vi "geis.vi"(3 "Draw":T2(ring), 7 "DLLPath":path, 8 "error in (no error)":errorcluster, 9 "GEIS Parameters":T3={"Step_number"=0, "Initial_Current_step"=0.0, "vs_initial "=TRUE, "Final_Current_step"=0.001, "vs_final"=TRUE, "Duration_step"=1.0, "Record_every_dE"=0.1, "Record_every_dT"=0.1, "Initial_frequency"=100000.0, "sweep"=FALSE, "Final_frequency"=1.0, "Frequency_number"=51, "Amplitude_Current"=0.001, "Wait_for_steady"=2.0, "Average_N_times"=1, "Correction"=TRUE, "I_Range"=7, "Bandwidth"=5, "em"=1, "ce"=0} {"ce" items=["Standard", "CE to ground"]; "em" max=10 format="%.5f"; "Initial_Current_step" min=-10 max=10 format="%.5f"; "Step_number" min=0 step=1; "I_Range" items=["1pA", "1nA", "10nA", "100nA", "1µA", "10µA", "100µA", "1mA", "10mA", "100mA", "1A", "Booster", "Auto"]; "Bandwidth" items=["1"=1, "2"=2, "3"=3, "4"=4, "5"=5, "6"=6, "7"=7, "8"=8, "9"=9]; "Wait_for_steady" min=0 format="%.2f"; "Record_every_dT" min=0 format="%.2e"; "Record_every_dE" min=0 format="%.2e"; "Duration_step" min=0 format="%.5f"; "Final_Current_step" min=-10 max=10 format="%.5f"; "Average_N_times" min=1 max=1000 step=1; "Amplitude_Current" min=0 max=100 format="%.2e"; "Final_frequency" min=1e-05 max=1000000 format="%.2e"; "Frequency_number" min=1 max=10000; "Initial_frequency" min=1e-05 max=1000000 format="%.2e"}, 10 "Channel":u8(ring) items=["1", "2", "3", "4", "5", "6", "7", "8", "9", "10", "11", "12", "13", "14", "15", "16"], 11 "IP adress":string="192.109.209.229") -> (0 "error out":errorcluster, 1 "OutputData":T1, 2 "Exit 2":bool=TRUE, 4 "XY Graph":cluster{"Data p1":sgl[], "Data p1":dbl[]}[](graph))   [LabVIEW 2022 SP3]
doc: "The Staircase Galvano Electrochemical Impedance Spectroscopy (SGEIS) technique is close to the SPEIS technique, except that the current is controlled instead of the potential.\n\nIn general, in this VI, the first thing to do is to start by establishing the connection with the instrument defined by its IP adress, then load the firmware in the channel selected, get the information on the plugged channels, load protocol on a channel, start/stop the protocol, retreive data and draw the graph.\nThis technique is applied just for channels with impedance capabilities (Zboard)."
uses:
  Library/EClib Functions/GEISParameters.ctl
  Library/EClib Functions/Parameters.ctl
  Library/EClib Functions/EClib functions.lvlib
panel:
  in  "Display Parameters?":bool caption="Display Parameters"
  out "DllPath":path caption="DLL Path"
  out "LibVersion":string caption="DLL Version"
  out "Data P0":sgl[][](array[numeric])=[[4.8e-05, 1.2033013, 0.0012545494], [7.2e-05, 4.099232, 0.0030298461], [9.6e-05, 5.4905596, 0.0034574724], [0.00040800002, 5.594096, 0.0031739129], [0.00086400006, 5.697314, 0.00286901], [0.0014160001, 5.800989, 0.0025610582], [0.002112, 5.903515, 0.002253106], [0.0030480002, 6.0050545, 0.0019497279], [0.0045120004, 6.105221, 0.0016379646], [0.008280001, 6.2053866, 0.0013155299], [0.100008, 6.222552, 0.0012118629], [0.200016, 6.223086, 0.0012103383], [0.300024, 6.223086, 0.0012126251], [0.400032, 6.2233143, 0.0012133875], [0.50004, 6.2231617, 0.0012141496], [0.600048, 6.2229333, 0.0012133875], [0.700056, 6.2229333, 0.0012103383], [0.800064, 6.2227044, 0.0012095761], [0.90007204, 6.2233143, 0.0012149118]]
  out "Data P1":sgl[][](array[numeric])=[[99999.99, 0.015896028, 2.4134535e-05, -0.31541085, 6.2027836, 0.0012093844, 0.0, 0.028001478, 2.4202996e-05, -0.21167731, -6.8013325, -0.001209385, 0.0, 1.296, 8.0], [79789.055, 0.020694803, 3.145496e-05, -0.31517792, 6.1967587, 0.0012085777, 0.0, 0.036134787, 3.1510877e-05, -0.20527963, -6.7949142, -0.0012085784, 0.0, 1.584, 8.0], [63671.867, 0.027115118, 3.95239e-05, -0.36039186, 6.1889963, 0.0012069115, 0.0, 0.04638151, 3.95688e-05, -0.23149349, -6.7864842, -0.0012069122, 0.0, 1.872, 8.0], [50804.684, 0.035882276, 4.949095e-05, -0.40444195, 6.178996, 0.0012048192, 0.0, 0.05973892, 4.952679e-05, -0.25926352, -6.77554, -0.0012048199, 0.0, 2.16, 8.0], [40539.06, 0.048188828, 6.136454e-05, -0.4440093, 6.1657524, 0.0012020994, 0.0, 0.077702746, 6.139315e-05, -0.28762102, -6.7610307, -0.0012021001, 0.0, 2.448, 8.0], [32343.752, 0.06770085, 7.88223e-05, -0.47251844, 6.1465006, 0.0011982684, 0.0, 0.10554845, 7.884587e-05, -0.31181583, -6.739913, -0.0011982691, 0.0, 2.736, 8.0], [25812.496, 0.12644306, 0.0001329111, -0.48514298, 6.0997047, 0.0011887155, 0.0, 0.19051811, 0.00013293685, -0.32698154, -6.6886125, -0.0011887162, 0.0, 3.024, 8.0], [20593.748, 0.23297587, 0.00022114319, -0.47706103, 6.015843, 0.0011718888, 0.0, 0.34030145, 0.00022117054, -0.3275948, -6.596549, -0.0011718895, 0.0, 3.312, 8.0], [16429.69, 0.37617812, 0.00032387703, -0.45101714, 5.8985395, 0.0011485365, 0.0, 0.5348972, 0.00032390282, -0.31515712, -6.4677424, -0.0011485372, 0.0, 3.6000001, 8.0], [13109.373, 0.55603534, 0.00044012873, -0.4103434, 5.7451816, 0.0011180385, 0.0, 0.7737537, 0.00044015126, -0.2906543, -6.299325, -0.0011180392, 0.0, 3.888, 8.0], [10460.936, 0.7749276, 0.00057313335, -0.36184657, 5.5526934, 0.001079828, 0.0, 1.0605142, 0.0005731519, -0.25886726, -6.0878835, -0.0010798287, 1.0, 4.176, 8.0], [8351.5625, 1.0352163, 0.00072714745, -0.31150156, 5.3164287, 0.0010371187, 1.0, 1.3994575, 0.0007271621, -0.22451091, -5.8299828, -0.0010371194, 1.0, 4.609, 8.0], [6660.1553, 1.3410046, 0.000907536, -0.26282227, 5.0436444, 0.0009789959, 1.0, 1.7970788, 0.00090754736, -0.19028175, -5.5293727, -0.0009789965, 2.0, 4.947, 8.0], [5313.953, 1.5113798, 0.0009967732, -0.21961367, 4.8940244, 0.0009556693, 1.0, 2.0129824, 0.000996781, -0.15885389, -5.3671427, -0.00095566985, 2.0, 5.57, 8.0], [4241.786, 1.5454612, 0.0010015898, -0.18297291, 4.878454, 0.0009537674, 1.0, 2.0500069, 0.0010015944, -0.13264023, -5.3505425, -0.0009537679, 2.0, 6.213, 8.0], [3385.4163, 1.5790181, 0.0010115571, -0.153041, 4.8648095, 0.00095176516, 1.0, 2.0889149, 0.0010115607, -0.111195564, -5.3358197, -0.0009517657, 2.0, 6.857, 8.0], [2699.3184, 1.5802759, 0.0010046018, -0.1293776, 4.883166, 0.0009544167, 1.0, 2.0867875, 0.0010046042, -0.09421384, -5.3556128, -0.0009544172, 2.0, 7.501, 8.0], [2153.4448, 1.5856456, 0.001002952, -0.11168504, 4.8972144, 0.0009564839, 1.0, 2.0912726, 0.0010029528, -0.08150327, -5.370766, -0.0009564844, 2.0, 8.1449995, 8.0], [1717.748, 1.5895984, 0.0010019304, -0.09921706, 4.9112163, 0.0009589054, 1.0, 2.0948448, 0.0010019315, -0.072561264, -5.38597, -0.0009589059, 2.0, 8.792, 8.0], [1372.1951, 1.5920151, 0.0010009218, -0.09178877, 4.924607, 0.0009613617, 1.0, 2.0966747, 0.0010009219, -0.06731814, -5.400561, -0.0009613622, 2.0, 9.439, 8.0], [1096.7545, 1.6009942, 0.0010047532, -0.08871567, 4.9333324, 0.000961253, 1.0, 2.1073825, 0.001004754, -0.06525302, -5.4094787, -0.00096125354, 2.0, 9.871, 8.0], [871.93097, 1.5816059, 0.0009906995, -0.09027839, 4.959241, 0.000966918, 1.0, 2.0806665, 0.0009906992, -0.06663093, -5.4381466, -0.00096691854, 2.0, 10.307, 8.0], [696.1138, 1.5729876, 0.0009832102, -0.09623489, 4.9737277, 0.0009698118, 1.0, 2.0679011, 0.0009832109, -0.07122159, -5.454079, -0.0009698124, 2.0, 10.741, 8.0], [555.8894, 1.6019666, 0.0009985057, -0.106960624, 4.9539285, 0.00096688373, 1.0, 2.1039863, 0.0009985064, -0.07941079, -5.4326506, -0.0009668843, 2.0, 11.394, 8.0], [443.43906, 1.6082691, 0.0009985616, -0.122988224, 4.9526095, 0.0009666943, 1.0, 2.1093283, 0.000998562, -0.091551304, -5.4311996, -0.00096669485, 2.0, 12.053, 8.0], [353.75473, 1.6163155, 0.0009975499, -0.14474046, 4.9489985, 0.00096599624, 1.0, 2.1154938, 0.0009975497, -0.10804355, -5.427236, -0.0009659968, 2.0, 12.715, 8.0], [281.8943, 1.6319947, 0.000997945, -0.1731171, 4.939253, 0.000964064, 1.0, 2.1291127, 0.0009979454, -0.12966967, -5.416549, -0.00096406456, 2.0, 13.377, 8.0], [225.3606, 1.6545873, 0.000997958, -0.20826769, 4.9249706, 0.00096138736, 1.0, 2.1484613, 0.0009979575, -0.15665877, -5.4009104, -0.0009613879, 2.0, 14.045, 8.0], [180.28844, 1.6867937, 0.0009969639, -0.25068158, 4.9050946, 0.0009575135, 1.0, 2.1753373, 0.0009969644, -0.18979812, -5.3791265, -0.0009575141, 2.0, 14.722, 8.0], [143.75787, 1.7397344, 0.0009973684, -0.30079174, 4.872224, 0.00095120573, 1.0, 2.2215395, 0.0009973678, -0.22964483, -5.3430943, -0.0009512063, 2.0, 15.411, 8.0], [114.59661, 1.8171204, 0.0009974693, -0.3567279, 4.8248806, 0.00094198145, 1.0, 2.2893379, 0.0009974696, -0.27555776, -5.2911463, -0.00094198197, 2.0, 16.109, 8.0], [91.552734, 1.9272654, 0.0009971086, -0.4146781, 4.7582307, 0.00092904264, 2.0, 2.3872557, 0.0009971082, -0.32522857, -5.217652, -0.00092904316, 2.0, 17.039999, 8.0], [72.87778, 2.0835702, 0.0009966118, -0.47080094, 4.6631265, 0.00091063714, 2.0, 2.5288415, 0.0009966121, -0.37639964, -5.1133604, -0.00091063767, 2.0, 17.782999, 8.0], [58.30223, 2.290216, 0.0009965424, -0.5163753, 4.536835, 0.00088618894, 2.0, 2.7210877, 0.000996542, -0.42156878, -4.9748783, -0.00088618946, 2.0, 18.546999, 8.0], [46.50297, 2.5567615, 0.0009965401, -0.54690737, 4.373813, 0.0008546952, 2.0, 2.9750876, 0.0009965405, -0.45663965, -4.796084, -0.00085469574, 2.0, 19.302, 8.0], [36.95101, 2.8818939, 0.0009962525, -0.55650496, 4.17603, 0.0008164121, 2.0, 3.292113, 0.0009962524, -0.47500235, -4.5792, -0.00081641256, 2.0, 20.077, 8.0], [29.592804, 3.234223, 0.0009962742, -0.5438912, 3.963954, 0.0007754039, 2.0, 3.6432135, 0.000996275, -0.47317147, -4.346668, -0.0007754044, 2.0, 20.93, 8.0], [23.588463, 3.6068342, 0.0009961284, -0.5106709, 3.7440598, 0.0007329593, 2.0, 4.0214486, 0.0009961289, -0.45162058, -4.1054997, -0.0007329597, 2.0, 21.862, 8.0], [18.780045, 3.9640598, 0.0009960186, -0.46161065, 3.5391219, 0.00069332117, 2.0, 4.3898535, 0.0009960192, -0.41360545, -3.8807545, -0.0006933216, 2.0, 22.863, 8.0], [15.024037, 4.271375, 0.0009959555, -0.40523124, 3.3689148, 0.00066039263, 2.0, 4.710784, 0.0009959557, -0.36663783, -3.694098, -0.00066039304, 2.0, 23.906, 8.0], [11.982363, 4.520932, 0.0009950611, -0.3458606, 3.2371411, 0.0006348915, 2.0, 4.9737754, 0.000995061, -0.31517577, -3.5495536, -0.0006348918, 2.0, 24.949, 8.0], [9.574144, 2.38077, 0.0005031747, -0.28917873, 4.6680098, 0.0009119648, 2.0, 2.6153588, 0.0005031747, -0.26482016, -5.1187296, -0.00091196527, 2.0, 25.382, 8.0], [7.6293964, 2.4353614, 0.0004999304, -0.23806715, 4.644746, 0.0009074361, 2.0, 2.6731777, 0.00049993006, -0.21878657, -5.0931625, -0.0009074366, 2.0, 25.922, 8.0], [6.084501, 2.4750657, 0.00049832056, -0.19374752, 4.6285977, 0.0009043441, 2.0, 2.7155764, 0.0004983205, -0.17844573, -5.075479, -0.0009043446, 2.0, 26.594, 8.0], [4.858519, 2.5030587, 0.0004974475, -0.15684187, 4.617654, 0.0009022134, 2.0, 2.7455964, 0.0004974477, -0.14467418, -5.0634913, -0.000902214, 2.0, 27.432001, 8.0], [3.8752477, 2.52257, 0.0004969658, -0.12630916, 4.6102643, 0.0009008552, 2.0, 2.7666035, 0.00049696607, -0.11720729, -5.055331, -0.00090085575, 2.0, 28.479, 8.0], [3.1001983, 2.5355425, 0.0004967685, -0.101694584, 4.6055255, 0.0008999815, 2.0, 2.7805579, 0.0004967687, -0.09457946, -5.050148, -0.000899982, 2.0, 29.784, 8.0], [2.4660668, 2.5443485, 0.00049676636, -0.0811795, 4.602378, 0.0008993778, 2.0, 2.7900364, 0.00049676653, -0.075683355, -5.046685, -0.0008993783, 2.0, 31.421001, 8.0], [1.9649143, 2.550054, 0.0004967066, -0.06482482, 4.600377, 0.0008989733, 2.0, 2.7961702, 0.0004967067, -0.060593843, -5.0444574, -0.00089897384, 2.0, 33.471, 8.0], [1.5725644, 2.5537558, 0.0004967495, -0.051944494, 4.599086, 0.00089873036, 2.0, 2.8001752, 0.0004967496, -0.04870844, -5.043045, -0.0008987309, 2.0, 36.029, 8.0], [1.2520034, 2.5562146, 0.00049671344, -0.04138118, 4.5982056, 0.00089857634, 2.0, 2.8028417, 0.00049671356, -0.03896928, -5.042108, -0.00089857687, 2.0, 39.239, 8.0], [1.0016024, 2.557709, 0.00049671053, -0.03315392, 4.597694, 0.0008984848, 2.0, 2.8044465, 0.00049671077, -0.031377077, -5.0415564, -0.00089848536, 2.0, 43.248, 8.0]]
  in  "stop":bool
  in  "Exit":bool
  in  "Start":bool
  out "Number of points":i32=52
  # "Instructions:\nBefore running the VI you must type a valid IP adress that corresponds to the instrument.Then press the Run button to execute this VI.\nWhile this VI is running, choose the available channel, enter the SGEIS parameters or keep the default\n values, then press the button start to begin the experience. \nChoose the waveform to draw : Nyquist, modZ, theta...\nPress the stop button to end experience and the exit button to stop the VI execution."
  # "Set I (A)  vs. previous"
  # "Before EIS  stay for ts (s)"
  # "and record every dE (V)"
  # "or every dt (s)"
  # "Start EIS from  Fi (Hz)"
  # "sweep linear/logarithmic"
  # "to Ff (Hz)"
  # "for Nf frequencies"
  # "with the amplitude (A)"
  # "wait for Pw"
  # "average Na times"
  # "drift correction"
  # "with I Range"
  # "bandwidth"
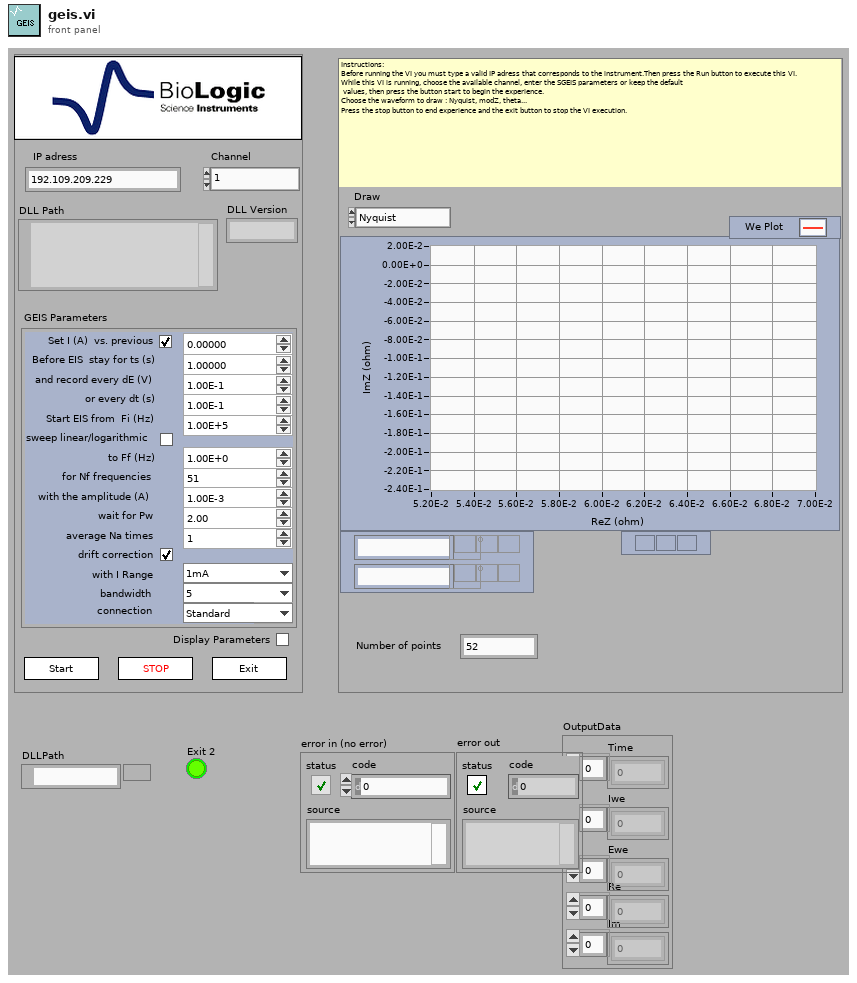
[diagram p1: front panel]
types:
  T1 = cluster{"Time":sgl[], "Iwe":sgl[], "Ewe":sgl[], "Re":sgl[], "Im":sgl[]}
  T2 = enum16{"Nyquist", "modZ", "theta", "modE", "modI", "Edc", "Idc", "E range", "I range", "f(t)", "Test"}
  T3 = typedef "EClib functions.lvlib/GEISParameters.ctl" = cluster{"Step_number":i32, "Initial_Current_step":sgl, "vs_initial ":bool, "Final_Current_step":sgl, "vs_final":bool, "Duration_step":sgl, "Record_every_dE":sgl, "Record_every_dT":sgl, "Initial_frequency":sgl, "sweep":bool, "Final_frequency":sgl, "Frequency_number":i32, "Amplitude_Current":sgl, "Wait_for_steady":sgl, "Average_N_times":i32, "Correction":bool, "I_Range":u16, "Bandwidth":u16, "em":u16, "ce":u16}
  T4 = cluster{"LibVersion":string, "StringLength":u32, "DllPath":path}
  T5 = cluster{"Channel":i32, "BoardVersion":i32, "BoardSerialCode":i32, "FirmwareCode":i32, "FirmwareVersion":i32, "XilinxVersion":i32, "AmpCode":i32, "NbAmp":i32, "LcBoard":i32, "Zboard":i32, "MuxBoard":i32, "GPRAboard":i32, "MemSize":i32, "MemFilled":i32, "state":i32, "MaxIRange":i32, "MinIRange":i32, "MaxBandwidth":i32, "NbOfTechniques":i32}
  T6 = typedef "EClib functions.lvlib/Parameters.ctl" = enum16{"CA", "CASG", "CP", "GEIS", "ISCAN", "OCV", "PEIS", "SCCX", "SGEIS", "SPEIS", "VSCAN", "MP"}
  T7 = typedef "EClib functions.lvlib/TechniqueParameters.ctl" = cluster{"String Label":string, "Type":i32, "Valeur":i32, "Index":i32}
  T8 = cluster{"string before end tag":string, i32, i32, i32}[]
  T9 = cluster{"IRQskipped":i32, "NbRaws":i32, "NbCols":i32, "Technique Index":i32, "TechniqueID":i32, "PrcessIndex":i32, "loop":i32, "StartTime":dbl, "MuxPad":i32}
  T10 = cluster{"State":i32, "MemFilled":i32, "TimeBase":sgl, " Ewe":sgl, " EweRangeMin":sgl, " EweRangeMax":sgl, "Ece":sgl, "EceRangeMin":sgl, "EceRangeMax":sgl, "Eoverflow":i32, "I":sgl, "IRange":i32, "Ioverflow":i32, "ElapsedTime":sgl, "Freq":sgl, "Rcomp":sgl, "Saturation":sgl, "OptErr":i32, "OptPos":i32}
  T11 = cluster{"Data P0":sgl[], "Data P0":sgl[], "Data P0":sgl[], sgl[], sgl[]}
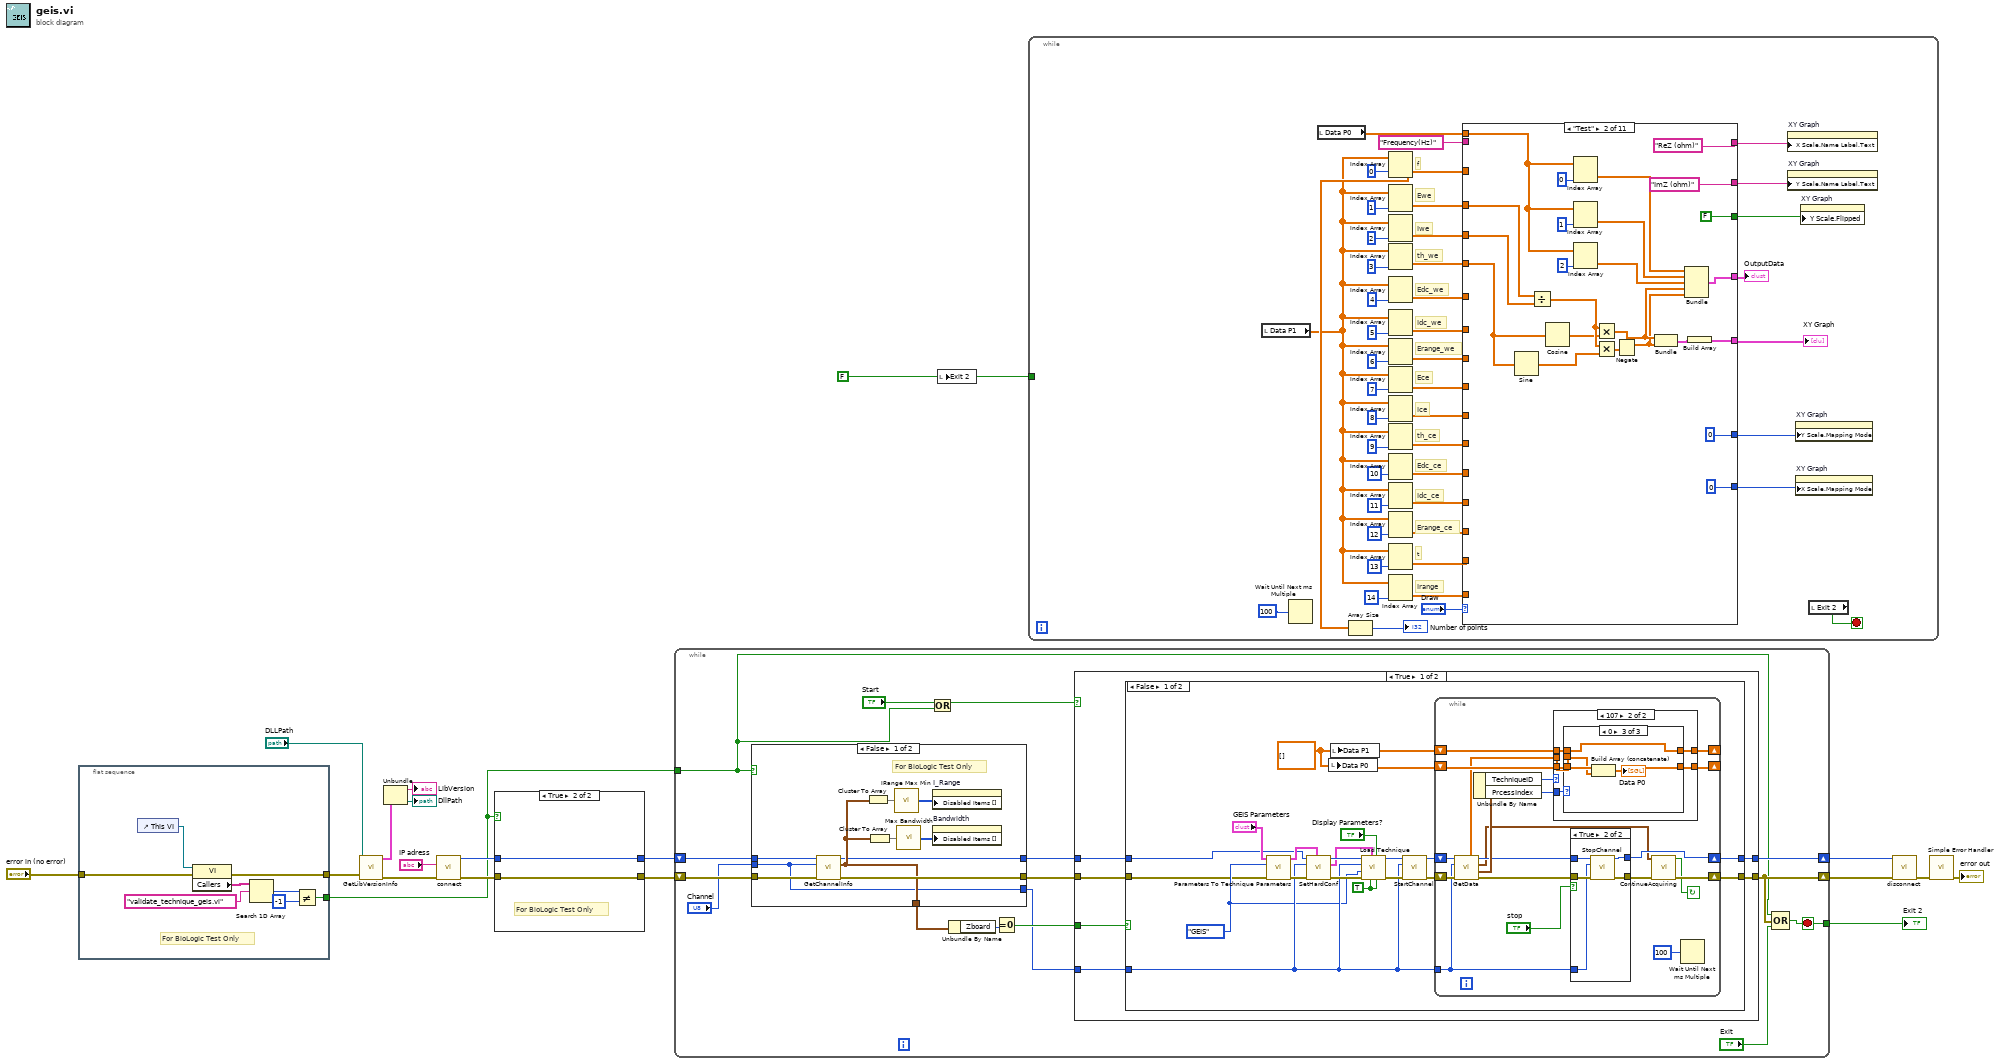
[diagram p0: block diagram]
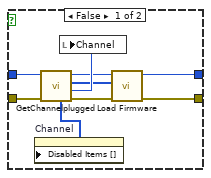
[diagram p2: hidden frame]
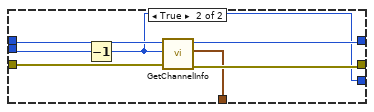
[diagram p3: hidden frame]
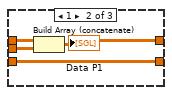
[diagram p6: hidden frame]
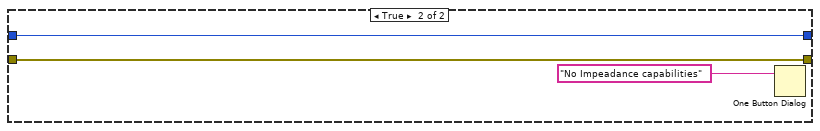
[diagram p8: hidden frame]
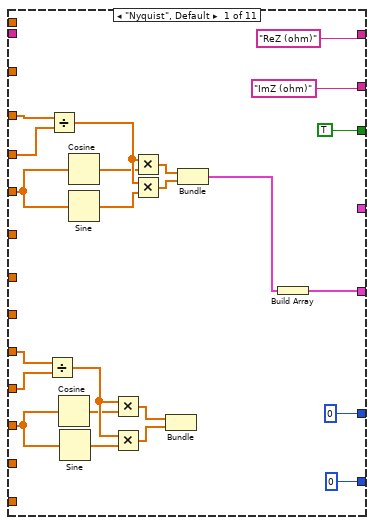
[diagram p10: hidden frame]
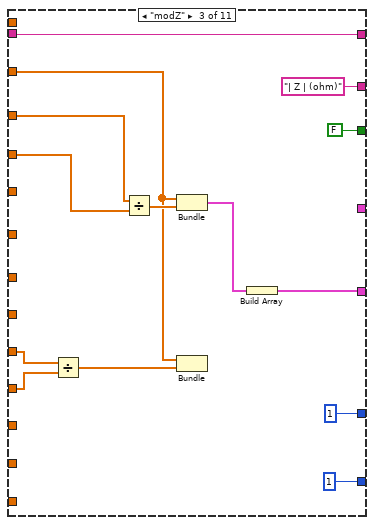
[diagram p11: hidden frame]
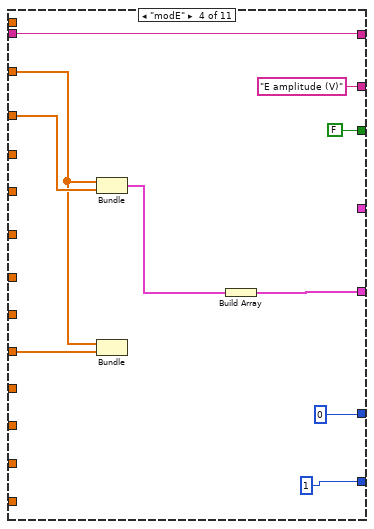
[diagram p12: hidden frame]
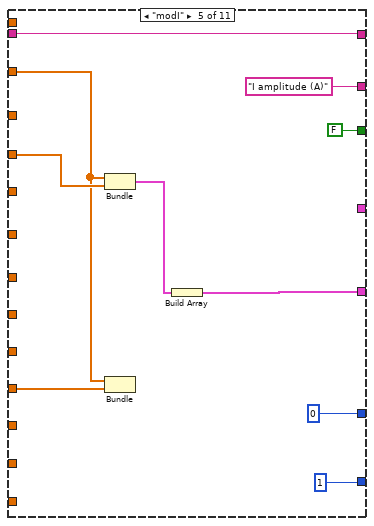
[diagram p13: hidden frame]
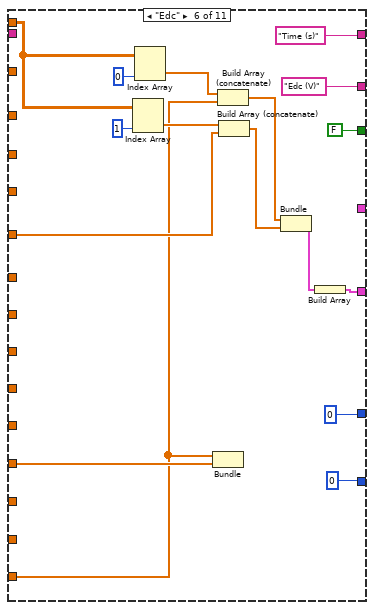
[diagram p14: hidden frame]
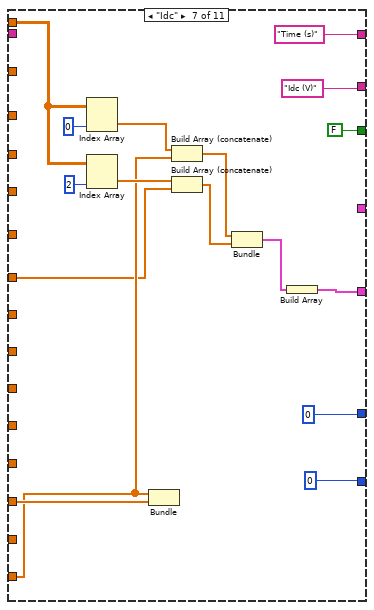
[diagram p15: hidden frame]
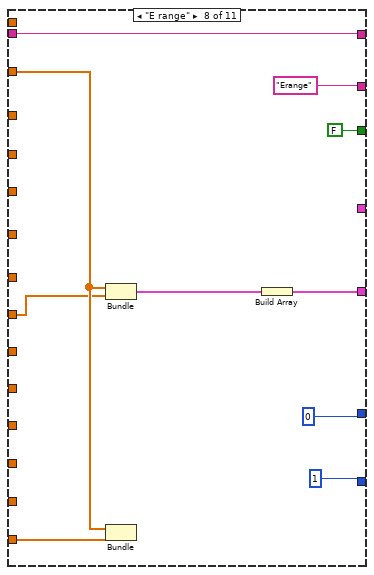
[diagram p16: hidden frame]
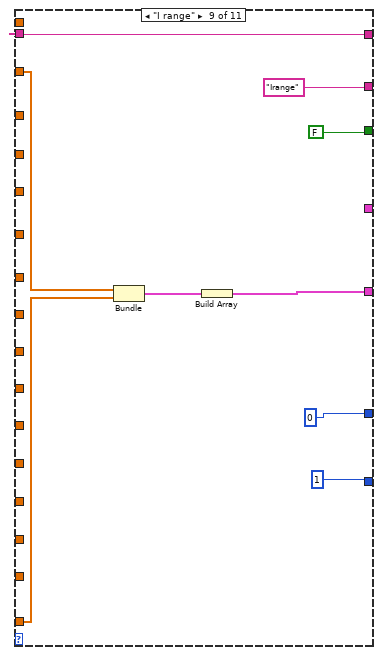
[diagram p17: hidden frame]
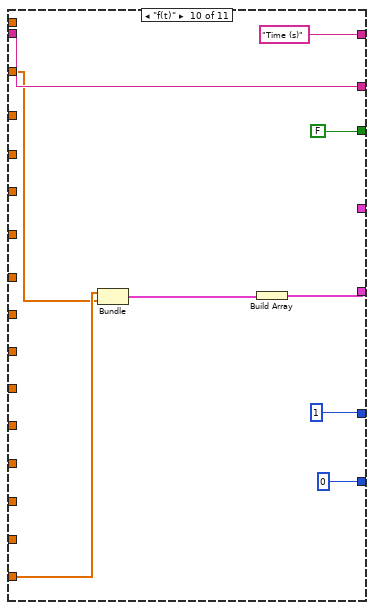
[diagram p18: hidden frame]
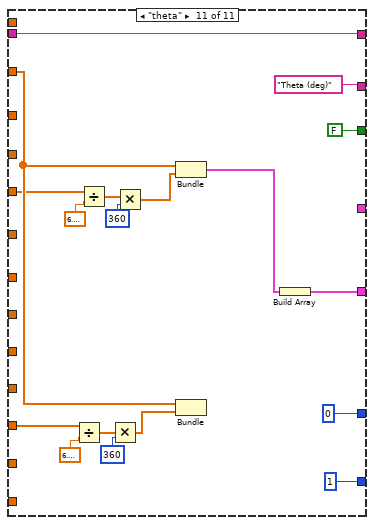
[diagram p19: hidden frame]
diagram:
  w18 = FALSE
  n1 = flat-sequence {
    tunnel: "error in (no error)" -> [w26]
    tunnel: [w21] -> w4
    tunnel: [w20] -> w5
    frame #0 {
      # "For BioLogic Test Only"
      n2 = control-ref of="This VI"() -> (w27:refnum<vi>)
      n3 = property class="VI"(reference=w27, error in=w26) -> (error out=w20:errorcluster, "Callers"=w25:string[])  [unwired: 1 out]
      n4 = Search 1D Array(1D array=w25, element="validate_technique_geis.vi") -> (index of element=w23:i32)  [unwired: 1 in]
      n5 = Not Equal?(x=w23, y=-1) -> (x != y?=w21:bool)
    }
  }
  n6 = call "GetLibVersionInfo.vi"("error in (no error)"=w5, "DLLPath"="DLLPath") -> ("error out"=w6:errorcluster, "LibInfo"=w9:T4)  [unwired: 8 in]
  n7 = Unbundle(w9) -> ("LibVersion"=→"LibVersion":string, "DllPath"=→"DllPath":path)  [unwired: 1 out]
  n8 = call "connect.vi"("error in (no error)"=w6, "IP"="IP adress") -> ("error out"=w14:errorcluster, "ID Out"=w16:i32)  [unwired: 5 in, 3 out]
  n9 = case shown="True" w4 {
    tunnel: w16 -> [w35 w38]
    tunnel: w14 -> [w34 w37]
    tunnel: [w32 w37] -> w13
    tunnel: [w30 w38] -> w12
    frame False {
      n10 = call "GetChannelplugged.vi"("error in (no error)"=w34, "ID In"=w35) -> ("error out"=w33:errorcluster, "FirstPluggedChannel"=w36:u8, "PluggedChannels"=w28:u8[], "ID Out"=w31:i32, "DisabledChannels"=w29:i32[])  [unwired: 5 in]
      n11 = property on="Channel" class="Ring (strict)"("Disabled Items []"=w29) -> ()  [unwired: 2 in, 2 out]
      n12 = local write "Channel"(w36) -> ()
      n13 = call "Load Firmware.vi"("error in (no error)"=w33, "Channels"=w28, "ID In"=w31) -> ("error out"=w32:errorcluster, "ID Out"=w30:i32)  [unwired: 6 in, 1 out]
    }
    frame True {
      # "For BioLogic Test Only"
    }
  }
  n14 = while {
    shift-right: [w44] -> w11
    shift-left: w13 -> [w50]
    tunnel: [w42] -> w17
    shift-right: [w51] -> w15
    shift-left: w12 -> [w46]
    tunnel: w4 -> [w39]
    stop <- w42 stop-if-true
    n15 = case shown="False" w39 {
      tunnel: w50 -> [w60 w71]
      tunnel: "Channel" -> [w55 w67]
      tunnel: [w59 w70] -> w48
      tunnel: [w58 w66] -> w47
      tunnel: w46 -> [w57 w69]
      tunnel: [w56 w68] -> w45
      tunnel: [w55 w65] -> w41
      frame False {
        # "For BioLogic Test Only"
        n16 = call "GetChannelInfo.vi"("error in (no error)"=w60, "Channel"=w55, "ID"=w57) -> ("error out"=w59:errorcluster, "Channel information"=w58:T5, "ID Out"=w56:i32)  [unwired: 6 in]
        n17 = Cluster To Array(cluster=w58) -> (array=w64:i32[])
        n18 = Cluster To Array(cluster=w58) -> (array=w63:i32[])
        n19 = call "IRange Max Min.vi"("resources"=w64) -> ("disabled ranges"=w61:i32[])
        n20 = call "Max Bandwidth.vi"("resources"=w63) -> ("disabled ranges"=w62:i32[])
        n21 = property on="I_Range" class="Ring (strict)"("Disabled Items []"=w61) -> ()  [unwired: 2 in, 2 out]
        n22 = property on="Bandwidth" class="Ring (strict)"("Disabled Items []"=w62) -> ()  [unwired: 2 in, 2 out]
      }
      frame True {
        n23 = Decrement(x=w67) -> (x-1=w65:u8)
        n24 = call "GetChannelInfo.vi"("error in (no error)"=w71, "Channel"=w65, "ID"=w69) -> ("error out"=w70:errorcluster, "Channel information"=w66:T5, "ID Out"=w68:i32)  [unwired: 6 in]
      }
    }
    n25 = Or(x="Start", y=w39) -> (x .or. y?=w40:bool)
    n26 = Unbundle By Name(w47) -> ("Zboard"=w53:i32)
    n27 = Equal To 0?(x=w53) -> (x = 0?=w52:bool)
    n28 = case shown="True" w40 {
      tunnel: w41 -> [w76 _]
      tunnel: [w77 w146] -> w44
      tunnel: w48 -> [w75 w146]
      tunnel: w52 -> [w74 _]
      tunnel: w45 -> [w73 w145]
      tunnel: [w72 w145] -> w51
      frame True {
        n29 = case shown="False" w74 {
          tunnel: [w96 w143] -> w77
          tunnel: w76 -> [w81 _]
          tunnel: w75 -> [w79 w143]
          tunnel: w73 -> [w78 w142]
          tunnel: [w88 w142] -> w72
          frame False {
            w80 = Parameters."GEIS" ("Parameters")
            w92 = TRUE ("First Protocol")
            w95 = sgl[][] [] ("Data")
            n30 = call "Parameters To Technique Parameters.vi"("error in (no error)"=w79, "Parameters"=w80, "ParameterIN"="GEIS Parameters") -> ("error out"=w87:errorcluster, "Params Values"=w84:T7[])  [unwired: 7 in]
            n31 = call "SetHardConf.vi"("Params Values"=w84, "error in (no error)"=w87, "Channel"=w81, "ID In"=w78) -> ("error out"=w86:errorcluster, "Params Values Trimed"=w83:T8, "ID Out"=w85:i32)  [unwired: 5 in]
            n32 = local write "Data P0"(w95) -> ()
            n33 = local write "Data P1"(w95) -> ()
            n34 = call "Load Technique.vi"("Last Protocol"=w92, "Display Parameters?"="Display Parameters?", "First Protocol"=w92, "TechniqueParameters"=w83, "error in (no error)"=w86, "Parameters"=w80, "Selected Channel"=w81, "ID In"=w85) -> ("error out"=w90:errorcluster, "ID  Out"=w91:i32)  [unwired: 1 in, 1 out]
            n35 = call "StartChannel.vi"("error in (no error)"=w90, "Channel"=w81, "ID In"=w91) -> ("error out"=w93:errorcluster, "ID Out"=w89:i32)  [unwired: 7 in]
            n36 = while {
              shift-right: [w102] -> w96
              shift-left: w93 -> [w115]
              shift-right: [w111] -> _
              shift-left: w95 -> [w112]
              shift-right: [w109] -> _
              shift-left: w95 -> [w110]
              shift-right: [w99] -> w88
              shift-left: w89 -> [w104]
              tunnel: w81 -> [w97]
              stop <- w100 continue-if-true
              n37 = call "GetData.vi"("error in (no error)"=w115, "Channel"=w97, "ID In"=w104) -> ("error out"=w113:errorcluster, "Data information"=w116:T9, "Current values"=w98:T10, "ID Out"=w103:i32, "Data"=w105:dbl[][])  [unwired: 1 in, 3 out]
              n38 = Unbundle By Name(w116) -> ("TechniqueID"=w107:i32, "PrcessIndex"=w106:i32)
              n39 = case shown="107" w107 {
                tunnel: w112 -> [w118 w124]
                tunnel: [w118 w123] -> w111
                tunnel: w110 -> [w117 w122]
                tunnel: [w117 w121] -> w109
                tunnel: w105 -> [_ w120]
                tunnel: w106 -> [_ w119]
                frame Default {
                }
                frame 107 {
                  n40 = case shown="0" w119 {
                    tunnel: [w126 w128 w131] -> w123
                    tunnel: w124 -> [w126 w129 w131]
                    tunnel: [w125 w127 w132] -> w121
                    tunnel: w122 -> [w125 w127 w134]
                    tunnel: w120 -> [_ w130 w133]
                    frame Default {
                    }
                    frame 1 {
                      n41 = Build Array (concatenate)(w129, w130) -> (w128:dbl[][])
                      "Data P1" <- w128
                    }
                    frame 0 {
                      n42 = Build Array (concatenate)(w134, w133) -> (w132:dbl[][])
                      "Data P0" <- w132
                    }
                  }
                }
              }
              n43 = case shown="True" "stop" {
                tunnel: [w136 w141] -> w101
                tunnel: w113 -> [w136 w140]
                tunnel: w103 -> [w135 w139]
                tunnel: [w135 w138] -> w99
                tunnel: w97 -> [_ w137]
                frame False {
                }
                frame True {
                  n44 = call "StopChannel.vi"("error in (no error)"=w140, "Channel"=w137, "ID In"=w139) -> ("error out"=w141:errorcluster, "ID Out"=w138:i32)  [unwired: 7 in]
                }
              }
              n45 = call "ContinueAcquiring.vi"("error in"=w101, "Current values"=w98) -> ("error out"=w102:errorcluster, "ContinueAcquiring?"=w100:bool)  [unwired: 8 in]
              n46 = Wait Until Next ms Multiple(millisecond multiple=u32 100) -> ()  [unwired: 1 out]
            }
          }
          frame True {
            n47 = One Button Dialog(message="No Impeadance capabilities" ("error source (\" \")")) -> ()  [unwired: 1 in, 1 out]
          }
        }
      }
      frame False {
      }
    }
    n48 = Compound Arithmetic op=OR(w39, w44, "Exit") -> (w42:bool)
  }
  "Exit 2" <- w17
  n49 = local write "Exit 2"(w18) -> ()
  n50 = while {
    tunnel: w18 -> [_]
    stop <- w179 stop-if-true
    # "Erange_ce"
    # "Idc_ce"
    # "Edc_ce"
    # "th_ce"
    # "Ice"
    # "Ece"
    # "t"
    # "Irange"
    # "Erange_we"
    # "Idc_we"
    # "Edc_we"
    # "th_we"
    # "Iwe"
    # "Ewe"
    # "f"
    n51 = local read "Data P1"() -> (w149:sgl[][])
    n52 = Wait Until Next ms Multiple(millisecond multiple=u32 100) -> ()  [unwired: 1 out]
    n53 = local read "Data P0"() -> (w148:sgl[][])
    n54 = Index Array(array=w149, index (col)=0 ("Index")) -> (element=w163:sgl[])  [unwired: 1 in]
    n55 = Array Size(array=w163) -> (size(s)=→"Number of points":i32)
    n56 = Index Array(array=w149, index (col)=1 ("Index")) -> (element=w164:sgl[])  [unwired: 1 in]
    n57 = Index Array(array=w149, index (col)=2 ("Index")) -> (element=w169:sgl[])  [unwired: 1 in]
    n58 = Index Array(array=w149, index (col)=3 ("Index")) -> (element=w184:sgl[])  [unwired: 1 in]
    n59 = Index Array(array=w149, index (col)=4 ("disabled index (col)")) -> (element=w178:sgl[])  [unwired: 1 in]
    n60 = Index Array(array=w149, index (col)=5 ("disabled index (col)")) -> (element=w175:sgl[])  [unwired: 1 in]
    n61 = Index Array(array=w149, index (col)=6 ("index (row)")) -> (element=w165:sgl[])  [unwired: 1 in]
    n62 = Index Array(array=w149, index (col)=7) -> (element=w156:sgl[])  [unwired: 1 in]
    n63 = Index Array(array=w149, index (col)=8) -> (element=w155:sgl[])  [unwired: 1 in]
    n64 = Index Array(array=w149, index (col)=9) -> (element=w154:sgl[])  [unwired: 1 in]
    n65 = Index Array(array=w149, index (col)=10) -> (element=w153:sgl[])  [unwired: 1 in]
    n66 = Index Array(array=w149, index (col)=11) -> (element=w152:sgl[])  [unwired: 1 in]
    n67 = Index Array(array=w149, index (col)=12) -> (element=w151:sgl[])  [unwired: 1 in]
    n68 = Index Array(array=w149, index (col)=13 ("disabled index (col)")) -> (element=w166:sgl[])  [unwired: 1 in]
    n69 = Index Array(array=w149, index (col)=14 ("disabled index (col)")) -> (element=w167:sgl[])  [unwired: 1 in]
    n70 = case shown="\"Test\"" "Draw" {
      tunnel: w163 -> [_ _ w244 w254 w265 _ _ w310 w318 w327 w338]
      tunnel: w164 -> [w196 w218 w242 w261 _ _ _ _ _ _ _]
      tunnel: w169 -> [w195 w217 w241 _ w271 _ _ _ _ _ _]
      tunnel: ["ImZ (ohm)" ("Y Scale.Name Label.Text") "ImZ (ohm)" ("Y Scale.Name Label.Text") "| Z | (ohm)" ("Y Scale.Name Label.Text") "E amplitude (V)" ("Y Scale.Name Label.Text") "I amplitude (A)" ("Y Scale.Name Label.Text") "Edc (V)" ("Y Scale.Name Label.Text") "Idc (V)" ("Y Scale.Name Label.Text") "Erange" ("Y Scale.Name Label.Text") "Irange" ("Y Scale.Name Label.Text") w332 "Theta (deg)" ("Y Scale.Name Label.Text")] -> w186
      tunnel: w184 -> [w191 w227 _ _ _ _ _ _ _ _ w336]
      tunnel: ["ReZ (ohm)" ("Y Scale.Name Label.Text") "ReZ (ohm)" ("Y Scale.Name Label.Text") w249 w259 w269 "Time (s)" ("Y Scale.Name Label.Text") "Time (s)" ("Y Scale.Name Label.Text") w315 w324 "Time (s)" ("Y Scale.Name Label.Text") w351] -> w183
      tunnel: "Frequency(Hz)" ("Y Scale.Name Label.Text") -> [_ _ w249 w259 w269 _ _ w315 w324 w332 w351]
      tunnel: [TRUE ("Y Scale.Flipped") FALSE ("Y Scale.Flipped") FALSE ("Y Scale.Flipped") FALSE ("Y Scale.Flipped") FALSE ("Y Scale.Flipped") FALSE ("Y Scale.Flipped") FALSE ("Y Scale.Flipped") FALSE ("Y Scale.Flipped") FALSE FALSE FALSE ("Y Scale.Flipped")] -> w181
      tunnel: [u8 0 ("X Scale.Mapping Mode") u8 0 ("X Scale.Mapping Mode") u8 1 ("X Scale.Mapping Mode") u8 1 ("X Scale.Mapping Mode") u8 1 ("X Scale.Mapping Mode") 0 0 1 1 0 u8 1 ("X Scale.Mapping Mode")] -> w180
      tunnel: w178 -> [_ _ _ _ _ w276 _ _ _ _ _]
      tunnel: w175 -> [_ _ _ _ _ _ w290 _ _ _ _]
      tunnel: w165 -> [_ _ _ _ _ _ _ w307 _ _ _]
      tunnel: w167 -> [_ _ _ _ _ _ _ _ w319 _ _]
      tunnel: w166 -> [_ _ _ _ _ w273 w291 _ _ w328 _]
      tunnel: [0 0 1 u8 0 ("X Scale.Mapping Mode") u8 0 ("X Scale.Mapping Mode") 0 0 0 0 1 0 ("X Scale.Mapping Mode")] -> w171
      tunnel: w156 -> [w194 _ w240 w255 _ _ _ _ _ _ _]
      tunnel: w155 -> [w193 _ w239 _ w264 _ _ _ _ _ _]
      tunnel: w154 -> [w192 _ _ _ _ _ _ _ _ _ w335]
      tunnel: w153 -> [_ _ _ _ _ w275 _ _ _ _ _]
      tunnel: w152 -> [_ _ _ _ _ _ w292 _ _ _ _]
      tunnel: w151 -> [_ _ _ _ _ _ _ w308 _ _ _]
      tunnel: [w201 w230 w238 w252 w262 w274 w293 w306 w316 w325 w334] -> w150
      tunnel: w148 -> [_ w223 _ _ _ w277 w294 _ _ _ _]
      tunnel: [_ w219 _ _ _ _ _ _ _ _ _] -> w147
      frame "Nyquist", Default {
        n71 = Divide(x=w194, y=w193) -> (x/y=w198:sgl[])
        n72 = Divide(x=w196, y=w195) -> (x/y=w200:sgl[])
        n73 = Cosine(x=w192) -> (cos(x)=w197:sgl[])
        n74 = Sine(x=w192) -> (sin(x)=w203:sgl[])
        n75 = Cosine(x=w191) -> (cos(x)=w199:sgl[])
        n76 = Sine(x=w191) -> (sin(x)=w213:sgl[])
        n77 = Multiply(x=w198, y=w197) -> (x*y=w205:sgl[])
        n78 = Multiply(x=w198, y=w203) -> (x*y=w204:sgl[])
        n79 = Multiply(x=w200, y=w199) -> (x*y=w207:sgl[])
        n80 = Multiply(x=w200, y=w213) -> (x*y=w208:sgl[])
        n81 = Bundle(w205, w204) -> ()  [unwired: 1 in, 1 out]
        n82 = Bundle(w207, w208) -> (w202:cluster{sgl[], sgl[]})  [unwired: 1 in]
        n83 = Build Array(w202) -> (w201:cluster{sgl[], sgl[]}[])
      }
      frame "Test" {
        n84 = Sine(x=w227) -> (sin(x)=w216:sgl[])
        n85 = Divide(x=w218, y=w217) -> (x/y=w229:sgl[])
        n86 = Cosine(x=w227) -> (cos(x)=w228:sgl[])
        n87 = Index Array(array=w223, index (col)=0 ("disabled index (col)")) -> (element=w222:sgl[])  [unwired: 1 in]
        n88 = Index Array(array=w223, index (col)=1 ("disabled index (col)")) -> (element=w221:sgl[])  [unwired: 1 in]
        n89 = Index Array(array=w223, index (col)=2 ("disabled index (col)")) -> (element=w220:sgl[])  [unwired: 1 in]
        n90 = Multiply(x=w229, y=w228) -> (x*y=w215:sgl[])
        n91 = Multiply(x=w229, y=w216) -> (x*y=w233:sgl[])
        n92 = Negate(x=w233) -> (-x=w214:sgl[])
        n93 = Bundle(w215, w214) -> (w231:cluster{sgl[], sgl[]})  [unwired: 1 in]
        n94 = Bundle("Data P0"=w222, "Data P0"=w221, "Data P0"=w220, w215, w214) -> (w219:T11)  [unwired: 1 in]
        n95 = Build Array(w231) -> (w230:cluster{sgl[], sgl[]}[])
      }
      frame "modZ" {
        n96 = Divide(x=w240, y=w239) -> (x/y=w245:sgl[])
        n97 = Divide(x=w242, y=w241) -> (x/y=w251:sgl[])
        n98 = Bundle("Data P1"=w244, w251) -> (w243:cluster{"Data P1":sgl[], sgl[]})  [unwired: 1 in]
        n99 = Bundle("Data P1"=w244, w245) -> ()  [unwired: 1 in, 1 out]
        n100 = Build Array(w243) -> (w238:cluster{"Data P1":sgl[], sgl[]}[])
      }
      frame "modE" {
        n101 = Bundle("Data P1"=w254, "Data P1"=w261) -> (w253:cluster{"Data P1":sgl[], "Data P1":sgl[]})  [unwired: 1 in]
        n102 = Bundle("Data P1"=w254, "Data P1"=w255) -> ()  [unwired: 1 in, 1 out]
        n103 = Build Array(w253) -> (w252:cluster{"Data P1":sgl[], "Data P1":sgl[]}[])
      }
      frame "modI" {
        n104 = Bundle("Data P1"=w265, "Data P1"=w271) -> (w263:cluster{"Data P1":sgl[], "Data P1":sgl[]})  [unwired: 1 in]
        n105 = Bundle("Data P1"=w265, "Data P1"=w264) -> ()  [unwired: 1 in, 1 out]
        n106 = Build Array(w263) -> (w262:cluster{"Data P1":sgl[], "Data P1":sgl[]}[])
      }
      frame "Edc" {
        n107 = Index Array(array=w277, index (col)=1 ("Index")) -> (element=w278:sgl[])  [unwired: 1 in]
        n108 = Index Array(array=w277, index (col)=0 ("Index")) -> (element=w279:sgl[])  [unwired: 1 in]
        n109 = Bundle("Data P1"=w273, "Data P1"=w275) -> ()  [unwired: 1 in, 1 out]
        n110 = Build Array (concatenate)(w279, w273) -> (w283:sgl[])
        n111 = Build Array (concatenate)(w278, w276) -> (w282:sgl[])
        n112 = Bundle(w283, w282) -> (w280:cluster{sgl[], sgl[]})  [unwired: 1 in]
        n113 = Build Array(w280) -> (w274:cluster{sgl[], sgl[]}[])
      }
      frame "Idc" {
        n114 = Index Array(array=w294, index (col)=0 ("Index")) -> (element=w298:sgl[])  [unwired: 1 in]
        n115 = Index Array(array=w294, index (col)=2 ("Index")) -> (element=w297:sgl[])  [unwired: 1 in]
        n116 = Bundle("Data P1"=w291, "Data P1"=w292) -> ()  [unwired: 1 in, 1 out]
        n117 = Build Array (concatenate)(w298, w291) -> (w296:sgl[])
        n118 = Build Array (concatenate)(w297, w290) -> (w295:sgl[])
        n119 = Bundle(w296, w295) -> (w301:cluster{sgl[], sgl[]})  [unwired: 1 in]
        n120 = Build Array(w301) -> (w293:cluster{sgl[], sgl[]}[])
      }
      frame "E range" {
        n121 = Bundle("Data P1"=w310, "Data P1"=w307) -> (w309:cluster{"Data P1":sgl[], "Data P1":sgl[]})  [unwired: 1 in]
        n122 = Bundle("Data P1"=w310, "Data P1"=w308) -> ()  [unwired: 1 in, 1 out]
        n123 = Build Array(w309) -> (w306:cluster{"Data P1":sgl[], "Data P1":sgl[]}[])
      }
      frame "I range" {
        n124 = Bundle("Data P1"=w318, "Data P1"=w319) -> (w317:cluster{"Data P1":sgl[], "Data P1":sgl[]})  [unwired: 1 in]
        n125 = Build Array(w317) -> (w316:cluster{"Data P1":sgl[], "Data P1":sgl[]}[])
      }
      frame "f(t)" {
        n126 = Bundle("Data P1"=w328, "Data P1"=w327) -> (w326:cluster{"Data P1":sgl[], "Data P1":sgl[]})  [unwired: 1 in]
        n127 = Build Array(w326) -> (w325:cluster{"Data P1":sgl[], "Data P1":sgl[]}[])
      }
      frame "theta" {
        n128 = Divide(x=w335, y=6.283185307179586) -> (x/y=w340:dbl[])
        n129 = Divide(x=w336, y=6.283185307179586) -> (x/y=w348:dbl[])
        n130 = Multiply(x=w340, y=360) -> (x*y=w342:dbl[])
        n131 = Multiply(x=w348, y=360) -> (x*y=w345:dbl[])
        n132 = Bundle("Data P1"=w338, w345) -> (w337:cluster{"Data P1":sgl[], dbl[]})  [unwired: 1 in]
        n133 = Bundle("Data P1"=w338, w342) -> ()  [unwired: 1 in, 1 out]
        n134 = Build Array(w337) -> (w334:cluster{"Data P1":sgl[], dbl[]}[])
      }
    }
    "XY Graph" <- w150
    "OutputData" <- w147
    n135 = property on="XY Graph" class="XYGraph (strict)"("X Scale.Name Label.Text"=w183) -> ()  [unwired: 2 in, 2 out]
    n136 = property on="XY Graph" class="XYGraph (strict)"("Y Scale.Name Label.Text"=w186) -> ()  [unwired: 2 in, 2 out]
    n137 = property on="XY Graph" class="XYGraph (strict)"("Y Scale.Mapping Mode"=w171) -> ()  [unwired: 2 in, 2 out]
    n138 = property on="XY Graph" class="XYGraph (strict)"("X Scale.Mapping Mode"=w180) -> ()  [unwired: 2 in, 2 out]
    n139 = property on="XY Graph" class="XYGraph (strict)"("Y Scale.Flipped"=w181) -> ()  [unwired: 2 in, 2 out]
    n140 = local read "Exit 2"() -> (w179:bool)
  }
  n141 = call "disconnect.vi"("error in (no error)"=w11, "ID In"=w15) -> ("error out"=w10:errorcluster)  [unwired: 9 in]
  n142 = call <vilib>:"Simple Error Handler.vi"("error in (no error)"=w10) -> ("error out"=→"error out":errorcluster)  [unwired: 4 in, 4 out]
